vi "Validate Field Name.vi"(8 "Error In":errorcluster, 11 "Field Name In":string) -> (0 "Error Out":errorcluster, 3 "Field Name Out":string)   [LabVIEW 2014, in "i3-sse-server.lvlib"]
uses:
  i3-sse-server.lvlib
  <vilib>/Utility/error.llb/Error Cluster From Error Code.vi
  <vilib>/ErrorRing/Error Ring.xnode
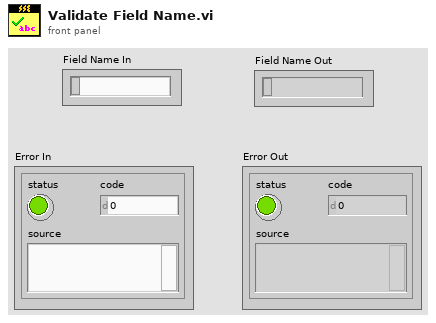
[diagram p1: front panel]
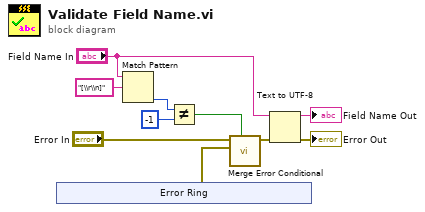
[diagram p0: block diagram]
diagram:
  n1 = xnode "Error Ring"() -> ("error out"=w7:errorcluster)
  n2 = Match Pattern(string="Field Name In", regular expression="[\\r\\n]") -> (offset past match=w8:i32)  [unwired: 1 in, 3 out]
  n3 = Not Equal?(x=w8, y=-1) -> (x != y?=w6:bool)
  n4 = call "Merge Error Conditional.vi"("Merge Error? (true)"=w6, "Error To Merge"=w7, "Original Error Wire"="Error In") -> ("Error Out"=w5:errorcluster)  [unwired: 8 in]
  n5 = Text to UTF-8(8:w5, 11:"Field Name In") -> (0:→"Error Out":errorcluster, 3:→"Field Name Out":string)  [unwired: 1 in]
